vi "aggregator - iii - real - atomic.vi"(6 "init?":bool, 7 "requested size":i32=20, 8 "number IN":dbl, 11 "state IN":T1={"Array "=[], "actual size"=0, "requested size"=20}) -> (0 "slope":dbl, 1 "interp average":dbl, 2 "mean":dbl, 3 "state OUT":T1={"Array "=[], "actual size"=0, "requested size"=20}, 4 "number OUT":dbl)   [LabVIEW 2021]
uses:
  interpolation state - real.ctl
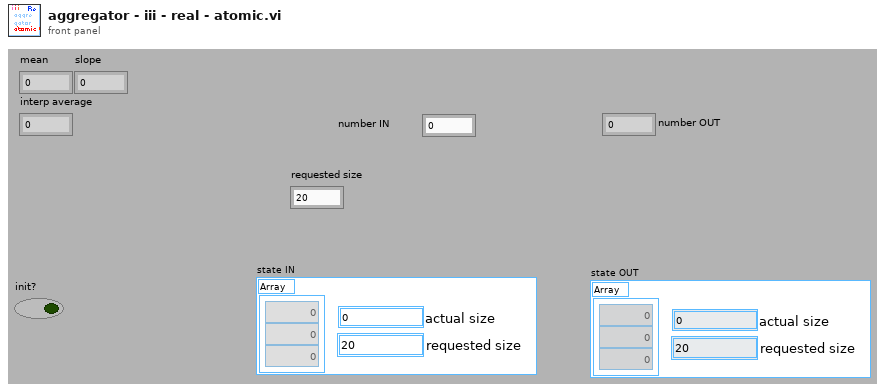
[diagram p1: front panel]
types:
  T1 = typedef "interpolation state - real.ctl" = cluster{"Array ":dbl[], "actual size":i32, "requested size":i32}
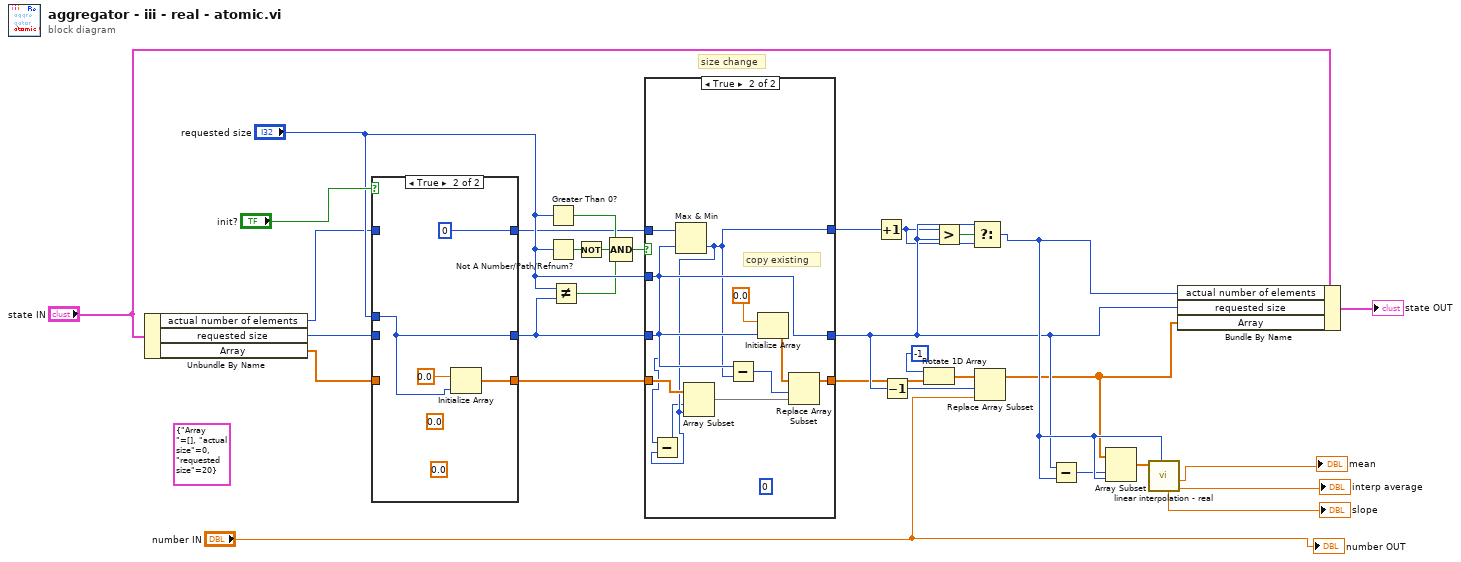
[diagram p0: block diagram]
diagram:
  (unwired) T1 {"Array "=[], "actual size"=0, "requested size"=20} ("Cluster")
  # "size change"
  n1 = Unbundle By Name("state IN") -> ("actual number of elements"=w25:i32, "requested size"=w26:i32, "Array"=w24:dbl[])
  n2 = case shown="True" "init?" {
    tunnel: w25 -> [w34 _]
    tunnel: [w34 0] -> w8
    tunnel: w24 -> [w32 _]
    tunnel: "requested size" -> [_ w35]
    tunnel: w26 -> [w33 _]
    tunnel: [w32 w36] -> w11
    tunnel: [w33 w35] -> w9
    frame False {
    }
    frame True {
      (unwired) 0.0
      (unwired) 0.0
      n3 = Initialize Array(0.0, w35) -> (w36:dbl[])
    }
  }
  n4 = Greater Than 0?(x="requested size") -> (x > 0?=w15:bool)
  n5 = Not A Number/Path/Refnum?(number/path/refnum="requested size") -> (NaN/Path/Refnum?=w16:bool)
  n6 = Not Equal?(x="requested size", y=w9) -> (x != y?=w13:bool)
  n7 = Not(x=w16) -> (.not. x?=w14:bool)
  n8 = Compound Arithmetic op=AND(w15, w14, w13) -> (w12:bool)
  n9 = case shown="True" w12 {
    tunnel: [w41 w43] -> w7
    tunnel: w8 -> [w41 w51]
    tunnel: [w40 w47] -> w20
    tunnel: w9 -> [w40 w44]
    tunnel: [w39 w50] -> w10
    tunnel: w11 -> [w39 w46]
    tunnel: "requested size" -> [_ w47]
    frame False {
    }
    frame True {
      (unwired) 0 ("disabled index (col)")
      # "copy existing"
      n10 = Max & Min(x=w51, y=w47) -> (min(x,y)=w43:i32)  [unwired: 1 out]
      n11 = Subtract(x=w44, y=w43) -> (x-y=w42:i32)
      n12 = Array Subset(array=w46, index=w42, length=w43) -> (w45:dbl[])
      n13 = Subtract(x=w47, y=w43) -> (x-y=w48:i32)
      n14 = Initialize Array(0.0, w47) -> (w49:dbl[])
      n15 = Replace Array Subset(array=w49, new element=w45, index=w48) -> (w50:dbl[])
    }
  }
  n16 = Increment(x=w7) -> (x+1=w17:i32)
  n17 = Decrement(x=w20) -> (x-1=w5:i32)
  n18 = Rotate 1D Array(1:w10, 2:-1 ("n")) -> (0:w4:dbl[])
  n19 = Greater?(x=w17, y=w20) -> (0:w18:bool)
  n20 = Select(t=w20, s=w18, f=w17) -> (s? t:f=w21:i32)
  n21 = Replace Array Subset(array=w4, new element="number IN", index=w5) -> (w19:dbl[])
  n22 = Subtract(x=w20, y=w21) -> (x-y=w3:i32)
  n23 = Array Subset(array=w19, index=w3, length=w21) -> (w2:dbl[])
  n24 = call "linear interpolation - real.vi"("n"=w21, "Array"=w2) -> ("interpolated average"=→"interp average":dbl, "mean"=→"mean":dbl, "slope"=→"slope":dbl)  [unwired: 4 in, 3 out]
  n25 = Bundle By Name(cluster="state IN", "actual number of elements"=w21, "requested size"=w20, "Array"=w19) -> (→"state OUT":T1)
  "number OUT" <- "number IN"
